vi "Teleop.vi"(8 "Call Context 2":T2=enum."Stop", 11 "Match Info 2":T1={"Autonomous Elapsed Seconds"=0.0, "TeleOp Elapsed Seconds"=171.498, "Disabled Elapsed Seconds"=31.356, "Visited Autonomous"=FALSE, "Visited TeleOp"=TRUE, "Visited Disabled"=TRUE, "Autonomous Settings"={"Autonomous Style"=enum."Independent", "VI Refnum"=refnum}}) -> ()   [LabVIEW 2012]
doc: "This VI is called for each TeleOp packet received from the DS where the robot is not disabled. It is often used to read from the joysticks and update I/O or to update setpoints for timed control loops. It should complete and return within 20 milliseconds or it may miss DS packets."
uses:
  <vilib>/Rock Robotics/WPI/DriverStation/WPI_DriverStationDerivedRobotMode.ctl
  <vilib>/Rock Robotics/WPI/DriverStation/WPI_DriverStationMatch Info.ctl
  Robot Global Data.vi
  <vilib>/Rock Robotics/WPI/Solenoid/Deprecated/WPI_SolenoidSetBool.vi
  <vilib>/Rock Robotics/WPI/RobotDrive/WPI_RobotDriveGetSetRefNum.vi
panel:
  # "The general plan for controlling the shooter is as follows:\nThe shooter can be controlled either manually or by a PID. As soon as Matt touches the joystick, he gets complete manual control, and must press a button to send control back to the PID.\nDepending on what is going on with the robot, the PID setpoint changes. It can be for going underneath the pyramid, climbing, recieving from the feeder station, moving up to shoot from the front\n of the pyramid, back of the pyramid, etc. When we get vision nailed down, we can use the vision code to automate the entire shooting operation.\n\nAn example of how this would work would be:\n1. Tyler takes control of the robot after autonomous, begins driving towards feeder station.\n2. Tyler presses buttons to raise uptake. Shooter automatically moves into position, belts start.\n3. Sensors detect 4 disks in shooter, shooter drops down to go under pyramid, belts stop, and uptake drops as well.\n4. Tyler drives under pyramid, someone presses button to raise shooter to shoot. \n5. Combination of vision/manual override get shooter into position.\n6. As soon as the first frisbee is fired, the belts start to push the one frisbee still in the belts into the hopper. \n7. When all four discs are fired, the shooter rotates down and tyler goes back to the feeder station, repeat.\n\nEndgame:\n1. A butto is pressed to raise shooter to climbing position, tyler drives into the pyramid.\n2. Limit switches on the hooks trip, stinger piston fires, leadscrews begin pulling down.\n3. When angle goes past a certain point, piston retracts and leadscrews stop.\n\nSome things to consider:\nCan we shoot 5 pointers? I don't see any reason why we can't except for difficulties lining up. A 20 point run would be much better than a 12 point run.\nWe need a sensor on the shooter wheel to detect speed. No more of this waiting/ overshooting buisness. Matt presses a button, the cam rotates as long as the shooter is up to speed. \nIf tyler engages feeder station, control is stripped from Matt."
  # "This is manual control of the shooter motor. The motor can turn so long as it stays between the upper and lower limits, unless button 5 (override) is pressed.\n Then it can go past the limits, possibly jamming the leadscrews"
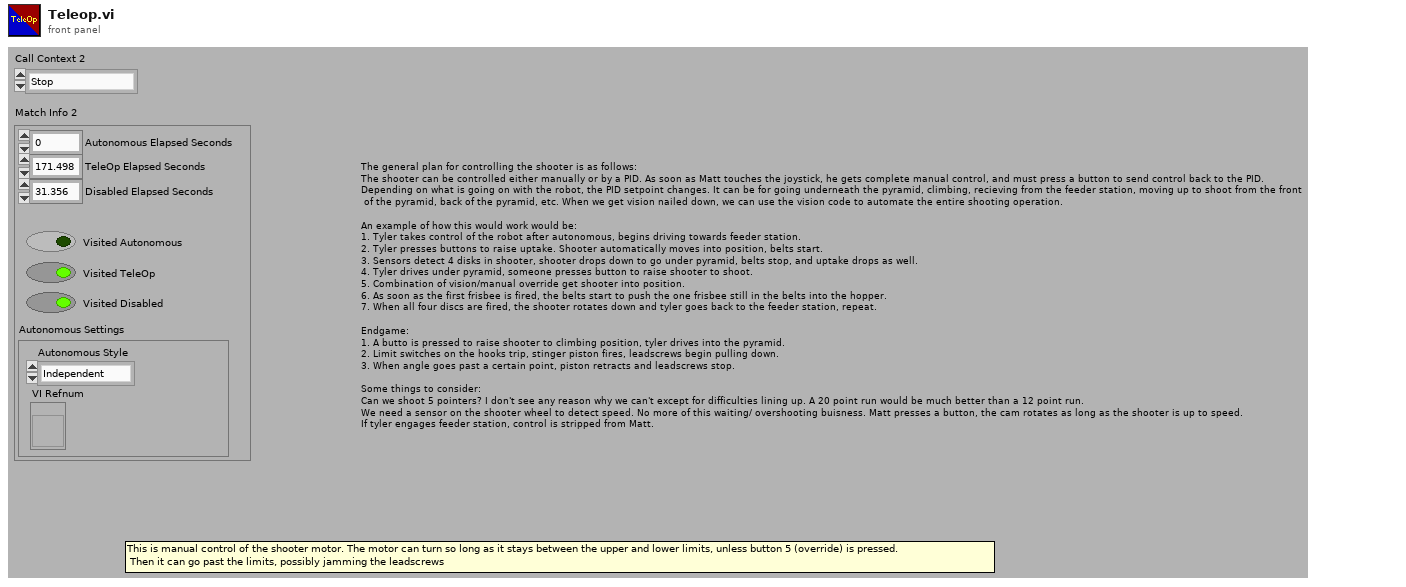
[diagram p1: front panel]
types:
  T1 = typedef "WPI_DriverStationMatch Info.ctl" = cluster{"Autonomous Elapsed Seconds":dbl, "TeleOp Elapsed Seconds":dbl, "Disabled Elapsed Seconds":dbl, "Visited Autonomous":bool, "Visited TeleOp":bool, "Visited Disabled":bool, "Autonomous Settings":cluster{"Autonomous Style":enum16{"Iterative", "Independent"}, "VI Refnum":refnum<vi>}}
  T2 = typedef "WPI_DriverStationDerivedRobotMode.ctl" = enum16{"Init", "Execute", "Stop"}
  T3 = typedef "WPI_RobotDriveDevRef.ctl" = cluster{"DevStatus":errorcluster, "Motors[]":T4[], "Square Inputs":bool, "Max Output":dbl, "Isochronous":bool}
  T4 = typedef "WPI_MotorControlDeviceRef.ctl" = cluster{"DeviceStatus":errorcluster, "Type":enum16{"PWM", "CAN"}, "PWM":cluster{"Digital Module":T5, "PWM Channel":T6, "DeadBand":T7}, "CAN":cluster{"Device Number":u8, "Control Mode":T8, "Semaphore":T9, "Max Vout":dbl}, "Invert":bool, "TransformRef":T10, "InvTransformRef":T10}
  T5 = typedef "FPGA_TypedefDigitalModule.ctl" = enum16{"Digital Module 1", "Digital Module 2"}
  T6 = typedef "FPGA_DIOPWMChannel.ctl" = enum8{"PWM 1", "PWM 2", "PWM 3", "PWM 4", "PWM 5", "PWM 6", "PWM 7", "PWM 8", "PWM 9", "PWM 10", "Invalid"}
  T7 = typedef "WPI_PWMDeadband.ctl" = cluster{"Name":string, "maxPositivePwm":i32, "minPositivePwm":i32, "centerPwm":i32, "maxNegativePwm":i32, "minNegativePwm":i32, "angularRange":u16}
  T8 = typedef "WPI_CANJaguar_ControlMode.ctl" = enum8{"Percent VBus", "Current", "Speed", "Position", "Voltage"}
  T9 = typedef "Semaphore RefNum" = refnum<k1>
  T10 = typedef "WPI_PWMTransform_ConPane.ctl" = refnum<vi>
  T11 = typedef "WPI_SolenoidDevRef.ctl" = cluster{"DevStatus":errorcluster, "Solenoid Module":T12, "Forward Solenoid Channel":T13, "Reverse Solenoid Channel":T13}
  T12 = typedef "FPGA_TypedefSolenoidModule.ctl" = enum16{"Solenoid Module 1", "Solenoid Module 2"}
  T13 = typedef "WPI_SolenoidChannel.ctl" = enum8{"Solenoid 1", "Solenoid 2", "Solenoid 3", "Solenoid 4", "Solenoid 5", "Solenoid 6", "Solenoid 7", "Solenoid 8", "Invalid"}
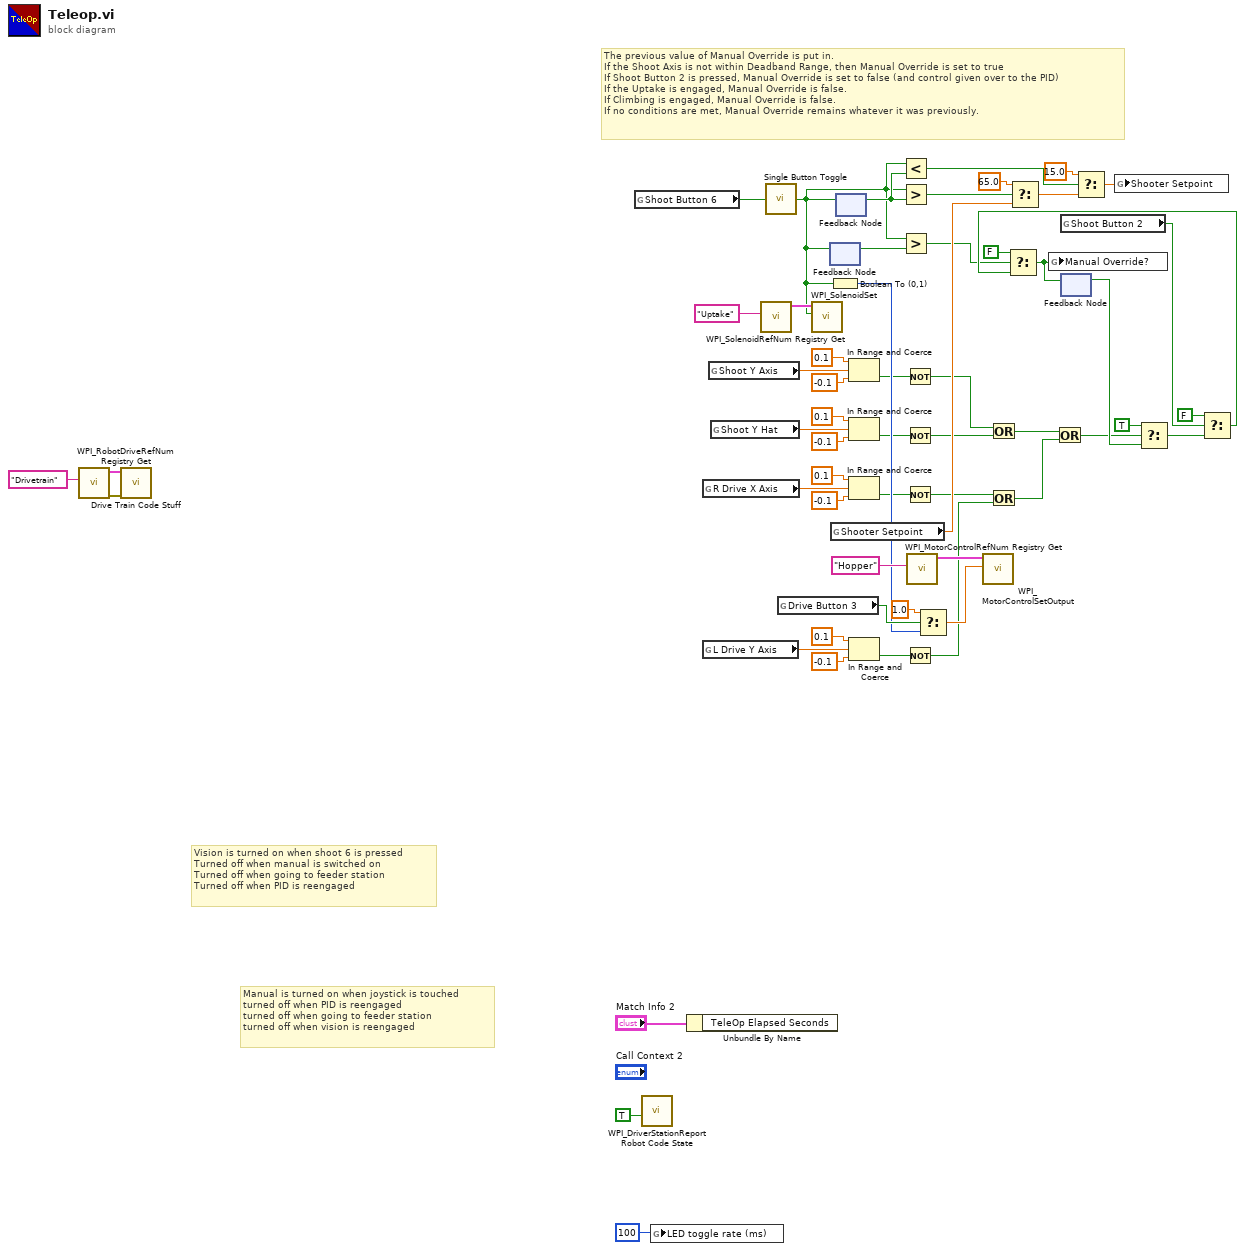
[diagram p0: block diagram]
diagram:
  # "Manual is turned on when joystick is touched\nturned off when PID is reengaged\nturned off when going to feeder station\nturned off when vision is reengaged"
  # "Vision is turned on when shoot 6 is pressed\nTurned off when manual is switched on\nTurned off when going to feeder station\nTurned off when PID is reengaged"
  # "The previous value of Manual Override is put in.\nIf the Shoot Axis is not within Deadband Range, then Manual Override is set to true\nIf Shoot Button 2 is pressed, Manual Override is set to false (and control given over to the PID)\nIf the Uptake is engaged, Manual Override is false.\nIf Climbing is engaged, Manual Override is false.\nIf no conditions are met, Manual Override remains whatever it was previously."
  n1 = call <vilib>:"WPI_RobotDriveRefNum Registry Get.vi"("refnum name"="Drivetrain") -> ("error out"=w50:errorcluster, "RobotDriveDevRef"=w51:T3)  [unwired: 1 in, 8 out]
  n2 = call "Drive Train Code Stuff.vi"("error in (no error)"=w50, "RobotDriveDevRef"=w51) -> ()  [unwired: 10 in]
  n3 = global read "Robot Global Data.vi" "Shoot Button 6"() -> (w28:bool)
  n4 = call <vilib>:"WPI_DriverStationReport Robot Code State.vi"("TeleOp"=TRUE ("Autonomous")) -> ()  [unwired: 10 in, 1 out]
  n5 = global write "Robot Global Data.vi" "LED toggle rate (ms)"(u32 100 ("LED ms toggle rate")) -> ()
  n6 = Unbundle By Name("Match Info 2") -> ()  [unwired: 1 out]
  n7 = global read "Robot Global Data.vi" "R Drive X Axis"() -> (w16:dbl)
  n8 = global read "Robot Global Data.vi" "L Drive Y Axis"() -> (w13:dbl)
  n9 = global read "Robot Global Data.vi" "Shoot Y Axis"() -> (w49:dbl)
  n10 = global read "Robot Global Data.vi" "Shoot Y Hat"() -> (w27:dbl)
  n11 = call <vilib>:"WPI_SolenoidRefNum Registry Get.vi"("refnum name"="Uptake") -> ("SolenoidDevRef"=w54:T11)  [unwired: 9 in, 1 out]
  n12 = call "Single Button Toggle.vi"("Shoot Button 3"=w28) -> ("Boolean"=w3:bool)
  n13 = global read "Robot Global Data.vi" "Drive Button 3"() -> (w34:bool)
  n14 = call-poly <vilib>:"WPI_SolenoidSet.vi"("Value"=w3, "SolenoidDevRef"=w54) -> ()  [unwired: 8 in, 2 out]
  n15 = feedback #1() -> (w2:bool)  [unwired: 1 in]
  n16 = feedback-in #1(w3) -> ()
  n17 = Boolean To (0,1)(Boolean=w3) -> (0, 1=w30:i16)
  n18 = global read "Robot Global Data.vi" "Shooter Setpoint"() -> (w43:dbl)
  n19 = feedback #2() -> (w39:bool)  [unwired: 1 in]
  n20 = feedback-in #2(w3) -> ()
  n21 = In Range and Coerce(upper limit=0.1, x=w49, lower limit=-0.1) -> (In Range?=w23:bool)  [unwired: 1 out]
  n22 = In Range and Coerce(upper limit=0.1, x=w27, lower limit=-0.1) -> (In Range?=w24:bool)  [unwired: 1 out]
  n23 = In Range and Coerce(upper limit=0.1, x=w16, lower limit=-0.1) -> (In Range?=w9:bool)  [unwired: 1 out]
  n24 = In Range and Coerce(upper limit=0.1, x=w13, lower limit=-0.1) -> (In Range?=w10:bool)  [unwired: 1 out]
  n25 = Less?(x=w3, y=w39) -> (x < y?=w38:bool)
  n26 = Greater?(x=w3, y=w39) -> (0:w40:bool)
  n27 = Greater?(x=w3, y=w2) -> (0:w1:bool)
  n28 = Not(x=w23) -> (.not. x?=w20:bool)
  n29 = Not(x=w24) -> (.not. x?=w19:bool)
  n30 = Not(x=w9) -> (.not. x?=w8:bool)
  n31 = Not(x=w10) -> (.not. x?=w7:bool)
  n32 = call <vilib>:"WPI_MotorControlRefNum Registry Get.vi"("refnum name"="Hopper") -> ("MotorControlDevRef"=w29:T4)  [unwired: 9 in, 1 out]
  n33 = Select(t=1.0, s=w34, f=w30) -> (s? t:f=w32:dbl)
  n34 = call <vilib>:"WPI_MotorControlSetOutput.vi"("Output"=w32, "MotorControlDevRef"=w29) -> ()  [unwired: 7 in, 3 out]
  n35 = Or(x=w20, y=w19) -> (x .or. y?=w6:bool)
  n36 = Or(x=w8, y=w7) -> (x .or. y?=w5:bool)
  n37 = Select(t=65.0 ("Uptake Setpoint"), s=w40, f=w43) -> (s? t:f=w37:dbl)
  n38 = Or(x=w6, y=w5) -> (x .or. y?=w4:bool)
  n39 = global read "Robot Global Data.vi" "Shoot Button 2"() -> (w41:bool)
  n40 = feedback #3() -> (w22:bool)  [unwired: 1 in]
  n41 = Select(t=15.0 ("Lower Setpoint"), s=w38, f=w37) -> (s? t:f=w18:dbl)
  n42 = global write "Robot Global Data.vi" "Shooter Setpoint"(w18) -> ()
  n43 = Select(t=TRUE ("f"), s=w4, f=w22) -> (s? t:f=w42:bool)
  n44 = Select(t=FALSE, s=w41, f=w42) -> (s? t:f=w45:bool)
  n45 = Select(t=FALSE, s=w1, f=w45) -> (s? t:f=w17:bool)
  n46 = global write "Robot Global Data.vi" "Manual Override?"(w17) -> ()
  n47 = feedback-in #3(w17) -> ()
